vi "ActualizarInventarioDBsql.vi"(8 "error in (no error)":errorcluster, 10 "INVENTARIO":i64, 11 "PRODUCTO":string) -> (0 "error out":errorcluster)   [LabVIEW 2020, in "DataBaseSQLlite.lvlib"]
uses:
  DataBaseSQLlite.lvlib
  <vilib>/drjdpowell/SQLite Library/SQL Connection/Open (path).vi
  <vilib>/drjdpowell/SQLite Library/SQL Connection/Open (string).vi
  <vilib>/AdvancedString/Path To Command Line String.vi
  <vilib>/drjdpowell/SQLite Library/SQL Connection/Execute SQL (No results).vi
  <vilib>/drjdpowell/SQLite Library/SQL Connection/Connection.lvclass
  <vilib>/drjdpowell/SQLite Library/SQLite.lvlib
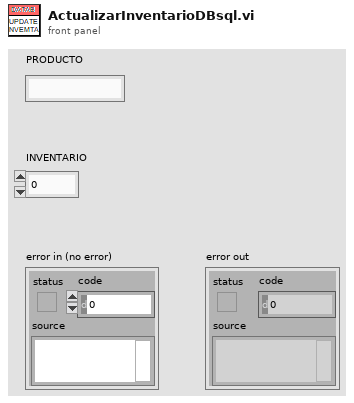
[diagram p1: front panel]
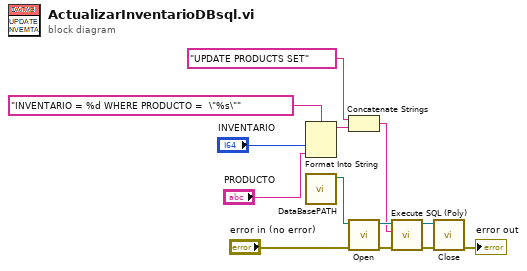
[diagram p0: block diagram]
diagram:
  n1 = Format Into String(format string="INVENTARIO = %d WHERE PRODUCTO =  \"%s\"", "INVENTARIO", "PRODUCTO") -> (resulting string=w12:string)  [unwired: 2 in, 1 out]
  n2 = call "DataBasePATH.vi"() -> ("DataBase path"=w10:path)  [unwired: 11 in]
  n3 = Concatenate Strings("UPDATE PRODUCTS SET" ("string"), w12) -> (w4:string)
  n4 = call-poly <vilib>:"Open.vi"("error in (no error)"="error in (no error)", "db file"=w10) -> ("error out"=w8:errorcluster, "SQLite Connection"=w9:refnum<class "Connection.lvclass">)  [unwired: 8 in]
  n5 = call-poly <vilib>:"Execute SQL (Poly).vi"("error in (no error)"=w8, "SQL"=w4, "SQLite Connection in"=w9) -> ("error out"=w6:errorcluster, "SQLite Connection"=w7:refnum<class "Connection.lvclass">)  [unwired: 7 in]
  n6 = call-dynamic "Close.vi"("error in (no error)"=w6, "SQLite Connection in"=w7) -> ("error out"=→"error out":errorcluster)  [unwired: 9 in]
